vi "Do.vi"(8 "error in (no error)":errorcluster, 10 "Actor in":refnum<class "Actor.lvclass">, 11 "EMS Device Activate Status Msg":refnum<class "EMS Device Activate Status Msg.lvclass">) -> (0 "error out":errorcluster, 2 "Actor out":refnum<class "Actor.lvclass">)   [LabVIEW 2015, in "Master Controller Core.lvlib" / "EMS Device Activate Status Msg.lvclass"]
doc: "This VI delivers the message to the actor by calling the appropriate method(s) on the actor."
uses:
  EMS Device Activate Status Msg.lvclass
  <vilib>/ActorFramework/Actor/Actor.lvclass
  Master Controller/Master Controller.lvclass
  SCADA Core/SCADA Abstract Messages/Device Action Status Msg/Device Action Status Msg.lvclass/Device Action Status Msg.ctl
  SCADA Core/SCADA Abstract Messages/Device Action Status Msg/Device Action Status Msg.lvclass
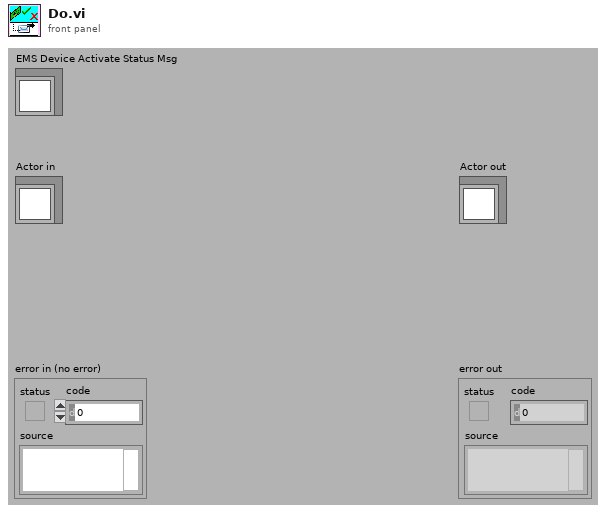
[diagram p1: front panel]
types:
  T1 = typedef "SCADA Core.lvlib/Device Action Status Msg.lvclass/Device Action Status.ctl" = enum16{"Success", "Failure"}
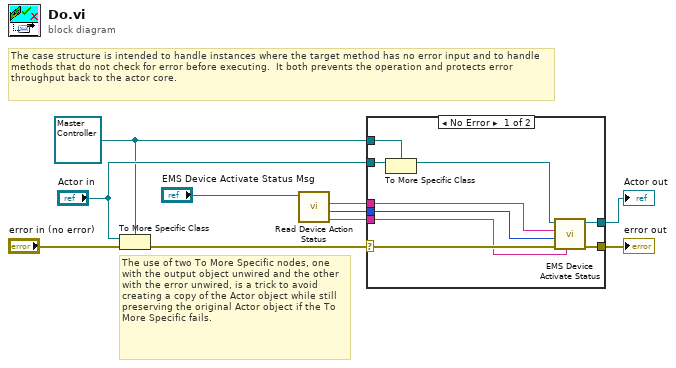
[diagram p0: block diagram]
diagram:
  w5 = refnum<class "Master Controller.lvclass"> refnum ("Actor in")
  # "The use of two To More Specific nodes, one with the output object unwired and the other with the error unwired, is a trick to avoid creating a copy of the Actor object while still preserving the original Actor object if the To More Specific fails."
  # "The case structure is intended to handle instances where the target method has no error input and to handle methods that do not check for error before executing.  It both prevents the operation and protects error throughput back to the actor core."
  n1 = To More Specific Class(target class=w5, reference="Actor in", error in="error in (no error)") -> (error out=w9:errorcluster)  [unwired: 1 out]
  n2 = call "Read Device Action Status.vi"("Island Control Status Msg in"="EMS Device Activate Status Msg") -> ("error string"=w1:string, "Status"=w2:T1, "IED Name"=w3:string)  [unwired: 7 in, 1 out]
  n3 = case shown="No Error" w9 {
    selector: w9 -> [w17 w21]
    tunnel: [w19 w21] -> w8
    tunnel: [w18 w20] -> w7
    tunnel: "Actor in" -> [w16 w20]
    tunnel: w5 -> [w15 _]
    tunnel: w3 -> [w13 _]
    tunnel: w2 -> [w12 _]
    tunnel: w1 -> [w11 _]
    frame No Error {
      n4 = To More Specific Class(target class=w15, reference=w16) -> (specific class reference=w14:refnum<class "Master Controller.lvclass">)  [unwired: 1 in, 1 out]
      n5 = call "EMS Device Activate Status.vi"("error string"=w11, "error in (no error)"=w17, "Status"=w12, "IED Name"=w13, "Master Controller in"=w14) -> ("error out"=w19:errorcluster, "Master Controller out"=w18:refnum<class "Master Controller.lvclass">)  [unwired: 5 in]
    }
    frame Error {
      # "If type check fails, pass the original object out again."
    }
  }
  "error out" <- w8
  "Actor out" <- w7
